vi "generate time clusters.vi"() -> (2 "origin times":T1[](array[typedef])=[{"day"=1, "hour"=5, "min"=11, "sec"=27, "msec"=34, "usec"=139, "nsec"=649}, {"day"=1, "hour"=5, "min"=11, "sec"=27, "msec"=33, "usec"=990, "nsec"=442}, {"day"=1, "hour"=5, "min"=11, "sec"=27, "msec"=34, "usec"=273, "nsec"=388}, {"day"=1, "hour"=5, "min"=11, "sec"=27, "msec"=33, "usec"=957, "nsec"=111}, {"day"=1, "hour"=5, "min"=11, "sec"=27, "msec"=34, "usec"=225, "nsec"=104}, {"day"=1, "hour"=5, "min"=11, "sec"=27, "msec"=33, "usec"=953, "nsec"=985}, {"day"=1, "hour"=5, "min"=11, "sec"=27, "msec"=34, "usec"=320, "nsec"=557}, {"day"=1, "hour"=5, "min"=11, "sec"=27, "msec"=33, "usec"=974, "nsec"=162}], 4 "position a times":T1[](array[typedef])=[{"day"=1, "hour"=5, "min"=11, "sec"=27, "msec"=37, "usec"=50, "nsec"=850}, {"day"=1, "hour"=5, "min"=11, "sec"=27, "msec"=36, "usec"=939, "nsec"=515}, {"day"=1, "hour"=5, "min"=11, "sec"=27, "msec"=37, "usec"=273, "nsec"=29}, {"day"=1, "hour"=5, "min"=11, "sec"=27, "msec"=37, "usec"=143, "nsec"=864}, {"day"=1, "hour"=5, "min"=11, "sec"=27, "msec"=37, "usec"=39, "nsec"=4}, {"day"=1, "hour"=5, "min"=11, "sec"=27, "msec"=37, "usec"=101, "nsec"=984}, {"day"=1, "hour"=5, "min"=11, "sec"=27, "msec"=37, "usec"=57, "nsec"=503}, {"day"=1, "hour"=5, "min"=11, "sec"=27, "msec"=37, "usec"=72, "nsec"=365}, {"day"=1, "hour"=5, "min"=11, "sec"=27, "msec"=37, "usec"=319, "nsec"=24}, {"day"=1, "hour"=5, "min"=11, "sec"=27, "msec"=37, "usec"=227, "nsec"=473}, {"day"=1, "hour"=5, "min"=11, "sec"=27, "msec"=37, "usec"=76, "nsec"=60}, {"day"=1, "hour"=5, "min"=11, "sec"=27, "msec"=37, "usec"=77, "nsec"=840}, {"day"=1, "hour"=5, "min"=11, "sec"=27, "msec"=37, "usec"=460, "nsec"=983}], 13 "position c times":T1[](array[typedef])=[{"day"=1, "hour"=5, "min"=11, "sec"=27, "msec"=35, "usec"=561, "nsec"=273}, {"day"=1, "hour"=5, "min"=11, "sec"=27, "msec"=35, "usec"=668, "nsec"=206}, {"day"=1, "hour"=5, "min"=11, "sec"=27, "msec"=35, "usec"=729, "nsec"=949}, {"day"=1, "hour"=5, "min"=11, "sec"=27, "msec"=35, "usec"=716, "nsec"=803}, {"day"=1, "hour"=5, "min"=11, "sec"=27, "msec"=35, "usec"=586, "nsec"=945}, {"day"=1, "hour"=5, "min"=11, "sec"=27, "msec"=35, "usec"=651, "nsec"=181}, {"day"=1, "hour"=5, "min"=11, "sec"=27, "msec"=35, "usec"=773, "nsec"=240}, {"day"=1, "hour"=5, "min"=11, "sec"=27, "msec"=35, "usec"=701, "nsec"=807}, {"day"=1, "hour"=5, "min"=11, "sec"=27, "msec"=35, "usec"=594, "nsec"=984}], 15 "position b times":T1[](array[typedef])=[{"day"=1, "hour"=5, "min"=11, "sec"=27, "msec"=36, "usec"=814, "nsec"=219}, {"day"=1, "hour"=5, "min"=11, "sec"=27, "msec"=36, "usec"=776, "nsec"=194}, {"day"=1, "hour"=5, "min"=11, "sec"=27, "msec"=36, "usec"=803, "nsec"=893}, {"day"=1, "hour"=5, "min"=11, "sec"=27, "msec"=36, "usec"=815, "nsec"=154}, {"day"=1, "hour"=5, "min"=11, "sec"=27, "msec"=36, "usec"=861, "nsec"=597}, {"day"=1, "hour"=5, "min"=11, "sec"=27, "msec"=36, "usec"=819, "nsec"=394}, {"day"=1, "hour"=5, "min"=11, "sec"=27, "msec"=36, "usec"=835, "nsec"=883}, {"day"=1, "hour"=5, "min"=11, "sec"=27, "msec"=36, "usec"=818, "nsec"=515}, {"day"=1, "hour"=5, "min"=11, "sec"=27, "msec"=36, "usec"=821, "nsec"=403}, {"day"=1, "hour"=5, "min"=11, "sec"=27, "msec"=36, "usec"=829, "nsec"=87}, {"day"=1, "hour"=5, "min"=11, "sec"=27, "msec"=36, "usec"=863, "nsec"=214}, {"day"=1, "hour"=5, "min"=11, "sec"=27, "msec"=36, "usec"=839, "nsec"=991}, {"day"=1, "hour"=5, "min"=11, "sec"=27, "msec"=36, "usec"=796, "nsec"=715}, {"day"=1, "hour"=5, "min"=11, "sec"=27, "msec"=36, "usec"=840, "nsec"=898}, {"day"=1, "hour"=5, "min"=11, "sec"=27, "msec"=36, "usec"=817, "nsec"=991}, {"day"=1, "hour"=5, "min"=11, "sec"=27, "msec"=36, "usec"=828, "nsec"=679}, {"day"=1, "hour"=5, "min"=11, "sec"=27, "msec"=36, "usec"=807, "nsec"=546}])   [LabVIEW 2014]
doc: "This subVI generates the four time cluster arrays for E4.\n\nPaul K Dixon\nP350\nCSUSB Physics"
uses:
  typedefs/time cluster typedef.ctl
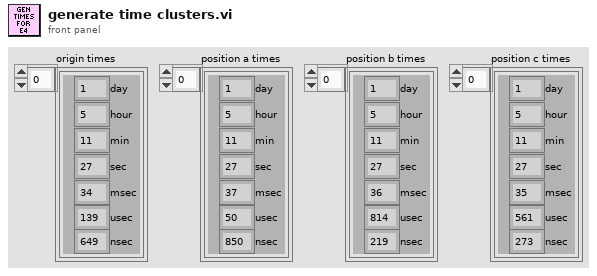
[diagram p1: front panel]
types:
  T1 = typedef "time cluster typedef.ctl" = cluster{"day":u32, "hour":u32, "min":u32, "sec":u32, "msec":u32, "usec":u32, "nsec":u32}
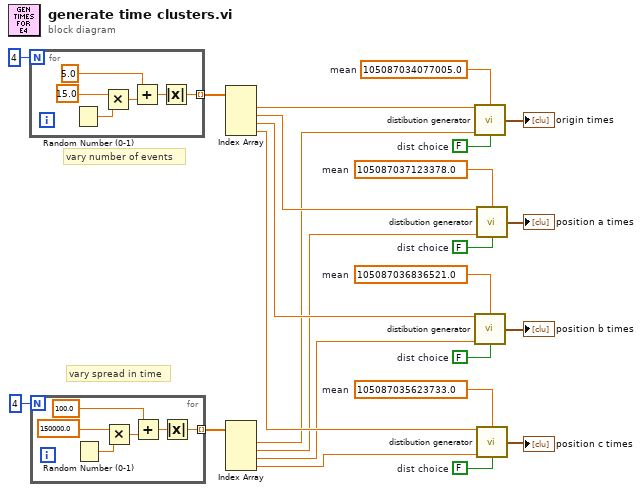
[diagram p0: block diagram]
diagram:
  w20 = FALSE  # dist choice
  w21 = 105087035623733.0  # mean
  w19 = FALSE  # dist choice
  w18 = 105087036836521.0  # mean
  w16 = FALSE  # dist choice
  w17 = 105087037123378.0  # mean
  w14 = FALSE  # dist choice
  w13 = 105087034077005.0  # mean
  # "vary spread in time"
  # "vary number of events"
  n1 = for {
    N: 4 -> [_]
    tunnel: [w25] -> w12 mode=indexing
    n2 = Random Number (0-1)() -> (number: 0 to 1=w30:dbl)
    n3 = Multiply(x=15.0, y=w30) -> (x*y=w29:dbl)
    n4 = Add(x=5.0, y=w29) -> (x+y=w28:dbl)
    n5 = Absolute Value(x=w28) -> (abs(x)=w25:dbl)
  }
  n6 = for {
    N: 4 -> [_]
    tunnel: [w31] -> w11 mode=indexing
    n7 = Random Number (0-1)() -> (number: 0 to 1=w36:dbl)
    n8 = Multiply(x=150000.0, y=w36) -> (x*y=w35:dbl)
    n9 = Add(x=100.0, y=w35) -> (x+y=w34:dbl)
    n10 = Absolute Value(x=w34) -> (abs(x)=w31:dbl)
  }
  n11 = Index Array(array=w12) -> (element #1=w10:dbl, element #2=w8:dbl, element #3=w7:dbl, element #4=w9:dbl)  [unwired: 4 in]
  n12 = Index Array(array=w11) -> (element #1=w3:dbl, element #2=w4:dbl, element #3=w5:dbl, element #4=w6:dbl)  [unwired: 4 in]
  n13 = call "distibution generator.vi"("samples"=w10, "mean (ns)"=w13, "standard deviation (ns)"=w3, "dist choice (T=flat/F=gauss)"=w14) -> ("time cluster array out"=→"origin times":T1[])  [unwired: 11 in]
  n14 = call "distibution generator.vi"("samples"=w7, "mean (ns)"=w18, "standard deviation (ns)"=w5, "dist choice (T=flat/F=gauss)"=w19) -> ("time cluster array out"=→"position b times":T1[])  [unwired: 11 in]
  n15 = call "distibution generator.vi"("samples"=w8, "mean (ns)"=w17, "standard deviation (ns)"=w4, "dist choice (T=flat/F=gauss)"=w16) -> ("time cluster array out"=→"position a times":T1[])  [unwired: 11 in]
  n16 = call "distibution generator.vi"("samples"=w9, "mean (ns)"=w21, "standard deviation (ns)"=w6, "dist choice (T=flat/F=gauss)"=w20) -> ("time cluster array out"=→"position c times":T1[])  [unwired: 11 in]
